vi "PID Run.vi"(5 "reinitialize? (F)":bool, 6 "manual control":dbl format="%.2f", 7 "auto? (T)":bool=TRUE, 8 "dt (s) in":dbl=-1.0, 9 "process variable":dbl step=0.01 format="%.2f", 10 "setpoint":dbl step=0.01 format="%.2f", 11 "PID in":refnum<class "PID.lvclass">) -> (0 "dt out (s)":dbl format="%.3f", 2 "output":dbl format="%.2f", 3 "PID out":refnum<class "PID.lvclass">)   [LabVIEW 2019, in "control.lvlib" / "PID.lvclass"]
uses:
  PID.lvclass
  D:/my_projects/projects/Algorithms/Labview/19/Reg/PID/PID Timing Estimation/PID Timing Estimation.lvclass
  PID Timing Estimation/PID Timing Estimation.lvclass/PID Timing Estimation.ctl
  PID.lvclass/PID.ctl
  PID Timing Estimation/PID Timing Estimation.lvclass
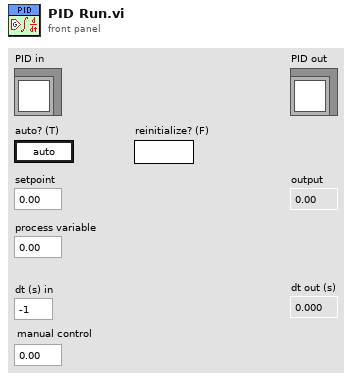
[diagram p1: front panel]
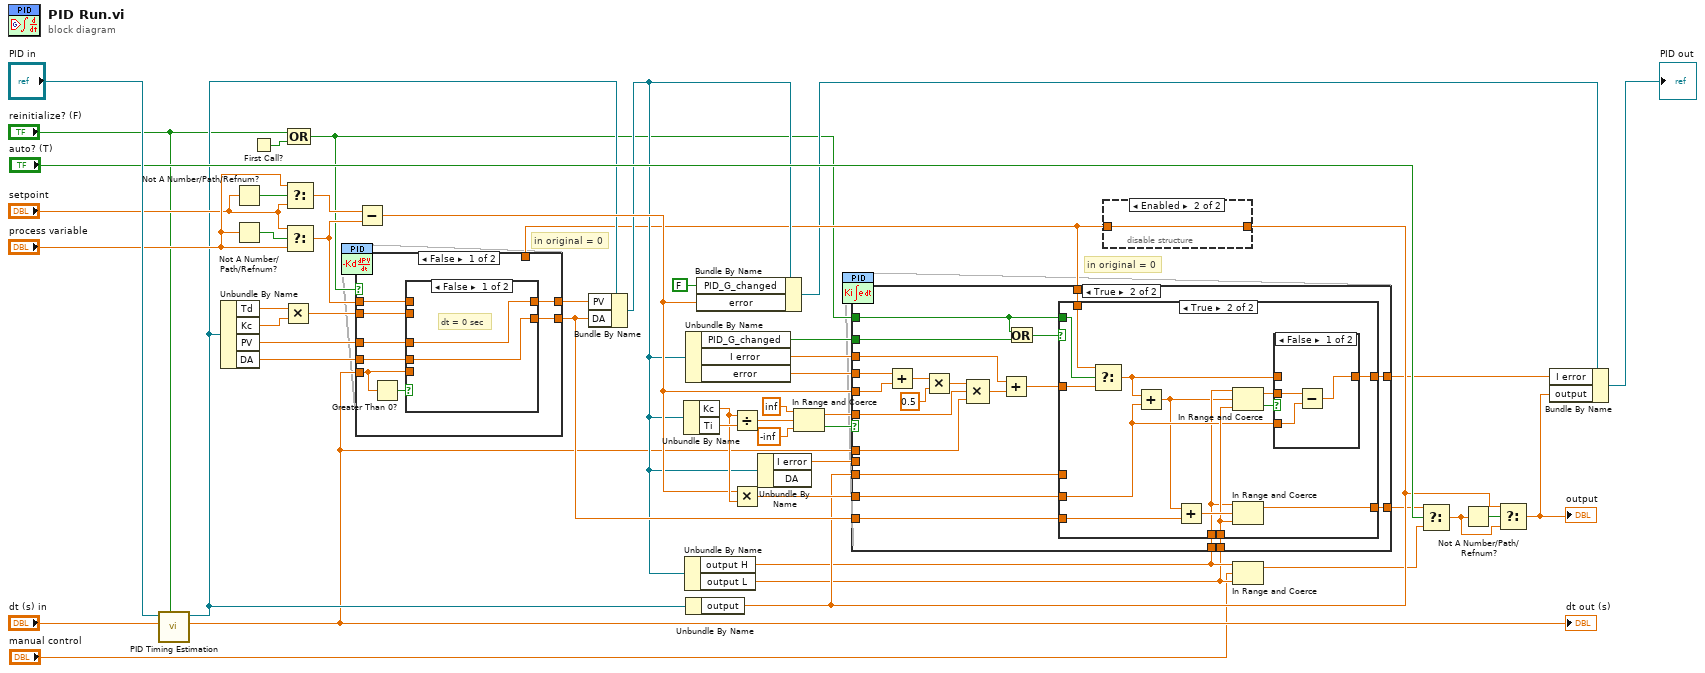
[diagram p0: block diagram]
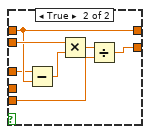
[diagram p2: hidden frame]
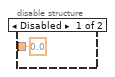
[diagram p4: hidden frame]
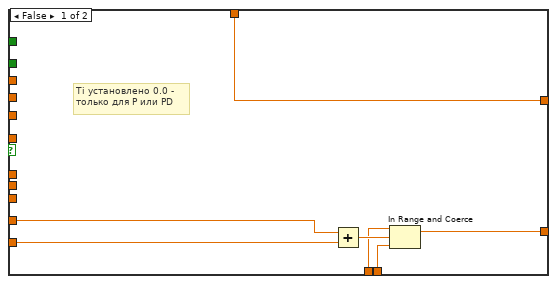
[diagram p5: hidden frame]
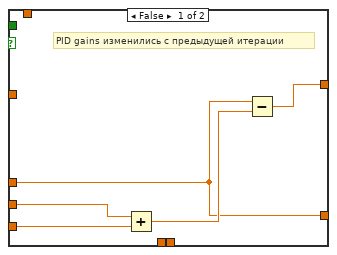
[diagram p6: hidden frame]
diagram:
  # "in original = 0"
  # "in original = 0"
  n1 = call "PID Timing Estimation.vi"("R"="reinitialize? (F)", "dt (s) in"="dt (s) in", "PID Timing Estimation in"="PID in") -> ("dt (s) out"=w5:dbl, "PID Timing Estimation out"=w16:refnum<class "PID.lvclass">)  [unwired: 7 in]
  "dt out (s)" <- w5
  n2 = Unbundle By Name(w16) -> ("Td"=w29:dbl, "Kc"=w32:dbl, "PV"=w31:dbl, "DA"=w28:dbl)
  n3 = Not A Number/Path/Refnum?(number/path/refnum="setpoint") -> (NaN/Path/Refnum?=w36:bool)
  n4 = Not A Number/Path/Refnum?(number/path/refnum="process variable") -> (NaN/Path/Refnum?=w37:bool)
  n5 = First Call?() -> (First Call?: T/F=w44:bool)
  n6 = Multiply(x=w29, y=w32) -> (x*y=w41:dbl)
  n7 = Select(t="process variable", s=w36, f="setpoint") -> (s? t:f=w35:dbl)
  n8 = Select(t="setpoint", s=w37, f="process variable") -> (s? t:f=w18:dbl)
  n9 = Compound Arithmetic op=OR("reinitialize? (F)", w44) -> (w11:bool)
  n10 = Subtract(x=w35, y=w18) -> (x-y=w19:dbl)
  n11 = Unbundle By Name(w16) -> ("output"=w14:dbl)
  n12 = disable-structure shown="Enabled" {
    disable-tunnel: [0.0 ("output") w51] -> w15
    disable-tunnel: w14 -> [_ w51]
    frame Disabled {
    }
    frame Enabled {
    }
  }
  n13 = case shown="False" w11 {
    tunnel: w31 -> [w59 _]
    tunnel: w41 -> [w56 _]
    tunnel: w18 -> [w58 w70]
    tunnel: [w55 w70] -> w25
    tunnel: [w57 w69] -> w24
    tunnel: w28 -> [w53 _]
    tunnel: w5 -> [w52 _]
    tunnel: w15 -> [_ w69]
    frame False {
      n14 = Greater Than 0?(x=w52) -> (x > 0?=w54:bool)
      n15 = case shown="False" w54 {
        tunnel: w59 -> [w61 w62]
        tunnel: w52 -> [_ w67]
        tunnel: w58 -> [_ w63]
        tunnel: [w60 w66] -> w57
        tunnel: w56 -> [_ w65]
        tunnel: [w61 w63] -> w55
        tunnel: w53 -> [w60 _]
        frame False {
          # "dt = 0 sec"
        }
        frame True {
          n16 = Subtract(x=w62, y=w63) -> (x-y=w64:dbl)
          n17 = Multiply(x=w65, y=w64) -> (x*y=w68:dbl)
          n18 = Divide(x=w68, y=w67) -> (x/y=w66:dbl)
        }
      }
    }
    frame True {
    }
  }
  n19 = Bundle By Name(cluster=w16, "PV"=w25, "DA"=w24) -> (w17:refnum<class "PID.lvclass">)
  n20 = Unbundle By Name(w17) -> ("Kc"=w23:dbl, "Ti"=w30:dbl)
  n21 = Unbundle By Name(w17) -> ("output H"=w4:dbl, "output L"=w3:dbl)
  n22 = Unbundle By Name(w17) -> ("PID_G_changed"=w22:bool, "I error"=w21:dbl, "error"=w27:dbl)
  n23 = Bundle By Name(cluster=w17, "PID_G_changed"=FALSE, "error"=w19) -> (w13:refnum<class "PID.lvclass">)
  n24 = Divide(x=w23, y=w30) -> (x/y=w40:dbl)
  n25 = Multiply(x=w19, y=w23) -> (x*y=w39:dbl)
  n26 = Unbundle By Name(w17) -> ("I error"=w26:dbl)  [unwired: 1 out]
  n27 = In Range and Coerce(upper limit=inf, x=w40, lower limit=-inf) -> (coerced(x)=w43:dbl, In Range?=w42:bool)
  n28 = case shown="True" w42 {
    tunnel: w27 -> [_ w97]
    tunnel: w19 -> [_ w98]
    tunnel: w26 -> [_ _]
    tunnel: [w71 w90] -> w12
    tunnel: w43 -> [_ w88]
    tunnel: w39 -> [w76 w93]
    tunnel: [w77 w89] -> w8
    tunnel: w14 -> [_ w91]
    tunnel: w24 -> [w75 w87]
    tunnel: w11 -> [_ w86]
    tunnel: w22 -> [_ w85]
    tunnel: w5 -> [_ w84]
    tunnel: w4 -> [w73 w82]
    tunnel: w3 -> [w72 w83]
    tunnel: w15 -> [w71 w81]
    tunnel: w21 -> [_ w78]
    frame False {
      # "Ti установлено 0.0 -\nтолько для P или PD"
      n29 = Add(x=w76, y=w75) -> (x+y=w74:dbl)
      n30 = In Range and Coerce(upper limit=w73, x=w74, lower limit=w72) -> (coerced(x)=w77:dbl)  [unwired: 1 out]
    }
    frame True {
      n31 = Add(x=w97, y=w98) -> (x+y=w96:dbl)
      n32 = Multiply(x=w96, y=0.5) -> (x*y=w95:dbl)
      n33 = Compound Arithmetic op=MULTIPLY(w95, w88, w84) -> (w79:dbl)
      n34 = Add(x=w78, y=w79) -> (x+y=w94:dbl)
      n35 = Or(x=w86, y=w85) -> (x .or. y?=w92:bool)
      n36 = case shown="True" w92 {
        tunnel: w94 -> [_ w104]
        tunnel: w93 -> [w102 w110]
        tunnel: w91 -> [w99 _]
        tunnel: w86 -> [_ w107]
        tunnel: [w103 w112] -> w90
        tunnel: [w99 w116] -> w89
        tunnel: w87 -> [w101 w115]
        tunnel: w83 -> [_ w114]
        tunnel: w82 -> [_ w109]
        tunnel: w81 -> [_ w106]
        frame False {
          # "PID gains изменились с предыдущей итерации"
          n37 = Add(x=w102, y=w101) -> (x+y=w100:dbl)
          n38 = Subtract(x=w99, y=w100) -> (x-y=w103:dbl)
        }
        frame True {
          n39 = Select(t=w106, s=w107, f=w104) -> (s? t:f=w105:dbl)
          n40 = Add(x=w105, y=w110) -> (x+y=w108:dbl)
          n41 = Add(x=w108, y=w115) -> (x+y=w117:dbl)
          n42 = In Range and Coerce(upper limit=w109, x=w108, lower limit=w114) -> (coerced(x)=w111:dbl, In Range?=w113:bool)
          n43 = In Range and Coerce(upper limit=w109, x=w117, lower limit=w114) -> (coerced(x)=w116:dbl)  [unwired: 1 out]
          n44 = case shown="False" w113 {
            tunnel: w105 -> [_ w121]
            tunnel: [w118 w121] -> w112
            tunnel: w111 -> [w120 _]
            tunnel: w110 -> [w119 _]
            frame False {
              n45 = Subtract(x=w120, y=w119) -> (x-y=w118:dbl)
            }
            frame True {
            }
          }
        }
      }
    }
  }
  n46 = In Range and Coerce(upper limit=w4, x="manual control", lower limit=w3) -> (coerced(x)=w1:dbl)  [unwired: 1 out]
  n47 = Select(t=w8, s="auto? (T)", f=w1) -> (s? t:f=w9:dbl)
  n48 = Not A Number/Path/Refnum?(number/path/refnum=w9) -> (NaN/Path/Refnum?=w38:bool)
  n49 = Select(t=w14, s=w38, f=w9) -> (s? t:f=w10:dbl)
  "output" <- w10
  n50 = Bundle By Name(cluster=w13, "I error"=w12, "output"=w10) -> (→"PID out":refnum<class "PID.lvclass">)
